vi "Tag.vi"(6 "Commit/Object":string, 7 "Tag Operation":T1, 8 "error in (no error)":errorcluster, 9 "Message":string, 10 "Tagname":string, 11 "Git Implementation in":refnum<class "Git Implementation.lvclass">) -> (0 "error out":errorcluster, 2 "Status Message":string, 3 "Git Implementation out":refnum<class "Git Implementation.lvclass">)   [LabVIEW 2017, in "Git-LabVIEW.lvlib" / "Git Implementation.lvclass"]
doc: "Create, list, delete or verify the signature of a tag object.\nBy default, use this VI to create annotated tags that can be pushed using Push together with the tags option.\nA signed tag requires a GnuPG key associated with your committer identity, found via your git-configuration.\nSee https://git-scm.com/docs/git-tag for further details."
uses:
  Git Implementation.lvclass
  Tag Operation.ctl
  <vilib>/Utility/error.llb/Error Cluster From Error Code.vi
  <vilib>/ErrorRing/Error Ring.xnode
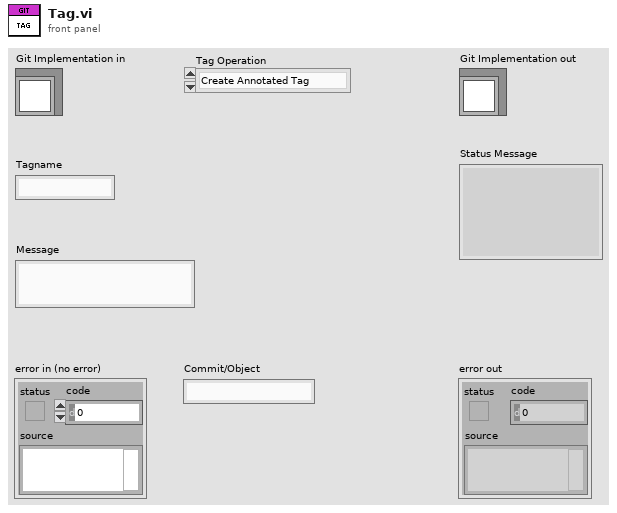
[diagram p1: front panel]
types:
  T1 = typedef "Git-LabVIEW.lvlib/Git Implementation.lvclass/Tag Operation.ctl" = enum16{"Create Annotated Tag", "Create Signed Tag", "List Tags", "Delete Tag", "Verify Tag"}
  T2 = typedef "Git-LabVIEW.lvlib/Git Implementation.lvclass/CMD Return.ctl" = cluster{"StdOut":string, "StdErr":string, "Return Code":i32}
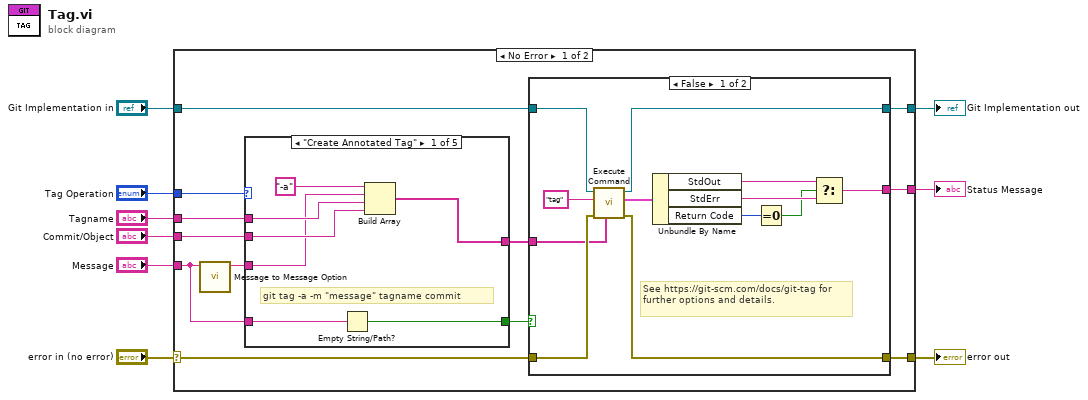
[diagram p0: block diagram]
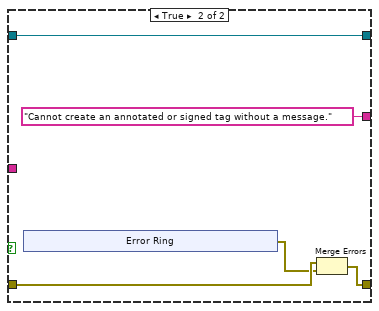
[diagram p2: hidden frame]
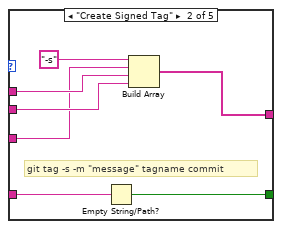
[diagram p3: hidden frame]
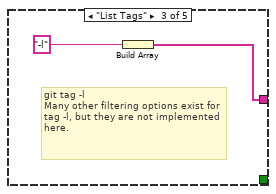
[diagram p4: hidden frame]
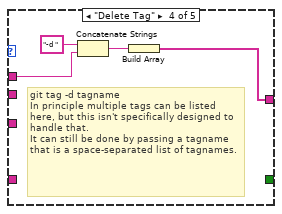
[diagram p5: hidden frame]
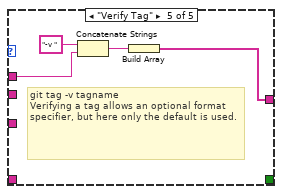
[diagram p6: hidden frame]
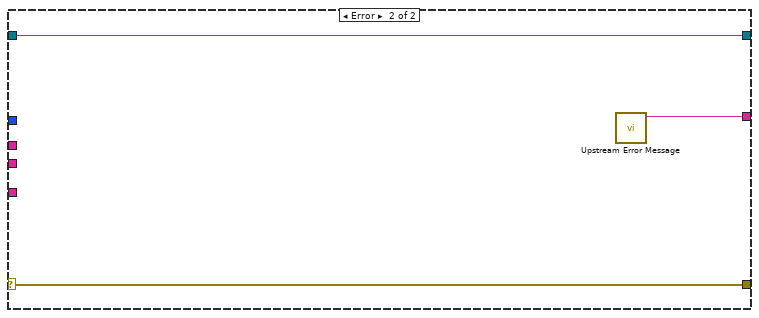
[diagram p7: hidden frame]
diagram:
  n1 = case shown="No Error" "error in (no error)" {
    selector: "error in (no error)" -> [w21 w69]
    tunnel: [w20 w69] -> w8
    tunnel: [w18 w68] -> w6
    tunnel: "Git Implementation in" -> [w19 w68]
    tunnel: "Message" -> [w10 _]
    tunnel: [w17 w67] -> w4
    tunnel: "Tag Operation" -> [w16 _]
    tunnel: "Tagname" -> [w13 _]
    tunnel: "Commit/Object" -> [w12 _]
    frame No Error {
      n2 = call "Message to Message Option.vi"("Message"=w10) -> ("Message Option"=w14:string)  [unwired: 10 in]
      n3 = case shown="\"Create Annotated Tag\"" w16 {
        tunnel: [w48 w55 w57 w61 w65] -> w15
        tunnel: w14 -> [w45 w52 _ _ _]
        tunnel: w13 -> [w47 w54 _ w59 w63]
        tunnel: w12 -> [w46 w53 _ _ _]
        tunnel: [w44 w51 _ _ _] -> w11
        tunnel: w10 -> [w43 w50 _ _ _]
        frame "Create Annotated Tag" {
          # "git tag -a -m \"message\" tagname commit"
          n4 = Empty String/Path?(string/path=w43) -> (empty?=w44:bool)
          n5 = Build Array("-a" ("Arguments"), w45, w47, w46) -> (w48:string[])
        }
        frame "Create Signed Tag" {
          # "git tag -s -m \"message\" tagname commit"
          n6 = Empty String/Path?(string/path=w50) -> (empty?=w51:bool)
          n7 = Build Array("-s" ("Arguments"), w52, w54, w53) -> (w55:string[])
        }
        frame "List Tags" {
          # "git tag -l\nMany other filtering options exist for tag -l, but they are not implemented here."
          n8 = Build Array("-l" ("Arguments")) -> (w57:string[])
        }
        frame "Delete Tag" {
          # "git tag -d tagname\nIn principle multiple tags can be listed here, but this isn't specifically designed to handle that.\nIt can still be done by passing a tagname that is a space-separated list of tagnames."
          n9 = Concatenate Strings("-d " ("Arguments"), w59) -> (w60:string)
          n10 = Build Array(w60) -> (w61:string[])
        }
        frame "Verify Tag" {
          # "git tag -v tagname\nVerifying a tag allows an optional format specifier, but here only the default is used."
          n11 = Concatenate Strings("-v " ("Arguments"), w63) -> (w64:string)
          n12 = Build Array(w64) -> (w65:string[])
        }
      }
      n13 = case shown="False" w11 {
        tunnel: w21 -> [w33 w36]
        tunnel: [w32 w35] -> w20
        tunnel: w19 -> [w30 w38]
        tunnel: [w29 w38] -> w18
        tunnel: [w23 "Cannot create an annotated or signed tag without a message." ("StdErr")] -> w17
        tunnel: w15 -> [w22 _]
        frame False {
          # "See https://git-scm.com/docs/git-tag for further options and details."
          n14 = call "Execute Command.vi"("Arguments"=w22, "error in (no error)"=w33, "Command"="tag", "Git Implementation in"=w30) -> ("error out"=w32:errorcluster, "CMD Return"=w28:T2, "Git Implementation out"=w29:refnum<class "Git Implementation.lvclass">)  [unwired: 5 in]
          n15 = Unbundle By Name(w28) -> ("StdOut"=w26:string, "StdErr"=w25:string, "Return Code"=w27:i32)
          n16 = Equal To 0?(x=w27) -> (x = 0?=w24:bool)
          n17 = Select(t=w26, s=w24, f=w25) -> (s? t:f=w23:string)
        }
        frame True {
          n18 = xnode "Error Ring"() -> ("error out"=w34:errorcluster)
          n19 = Merge Errors(w36, w34) -> (w35:errorcluster)
        }
      }
    }
    frame Error {
      n20 = call "Upstream Error Message.vi"() -> ("Upstream Error Message"=w67:string)  [unwired: 11 in]
    }
  }
  "error out" <- w8
  "Git Implementation out" <- w6
  "Status Message" <- w4
